vi "Init Control.vi"(5 "Group":refnum<class "Group DBL.lvclass">, 6 "Period ms":i64, 7 "VolatusAPI":refnum<class "VolatusAPI.lvclass">, 8 "error in (no error)":errorcluster, 9 "Control MsgQ":refnum<class "MessageQ.lvclass">, 10 "Config Element":refnum<class "Config Element.lvclass">, 11 "Valve in":refnum<class "LimitControl.lvclass">) -> (0 "error out":errorcluster, 3 "Valve out":refnum<class "LimitControl.lvclass">)   [LabVIEW 2020, in "VolatusControl.lvlib" / "LimitControl.lvclass"]
uses:
  LimitControl.lvclass
  lv-cdm/CDM-Config/Config Element/Config Element.lvclass
  Volatus/VolatusAPI/VolatusAPI.lvclass
  Volatus/MessageQ/MessageQ.lvclass
  lv-vecto/Vecto/Group DBL/Group DBL.lvclass
  C:/dev/lv20CE/relink/lv-vecto/Vecto/Group/Group.lvclass
  PV Calc.ctl
  LimitControl.lvclass/LimitControl.ctl
  lv-vecto/Vecto/Group/Group.lvclass
  VolatusControl.lvlib
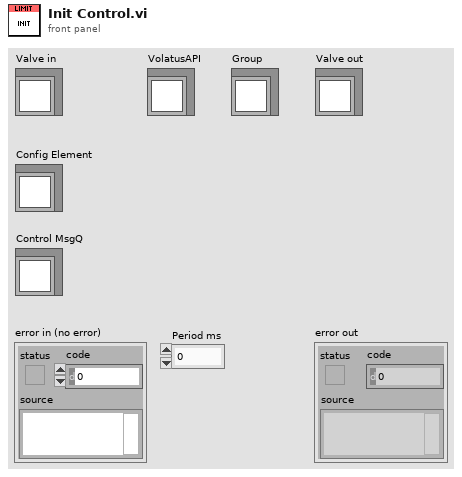
[diagram p1: front panel]
types:
  T1 = typedef "VolatusControl.lvlib/LimitControl.lvclass/PV Calc.ctl" = enum16{"Average", "Median"}
  T2 = typedef "CDM-Config.lvlib/Value Type.ctl" = enum16{"String", "Number", "Bool", "Object", "Array"}
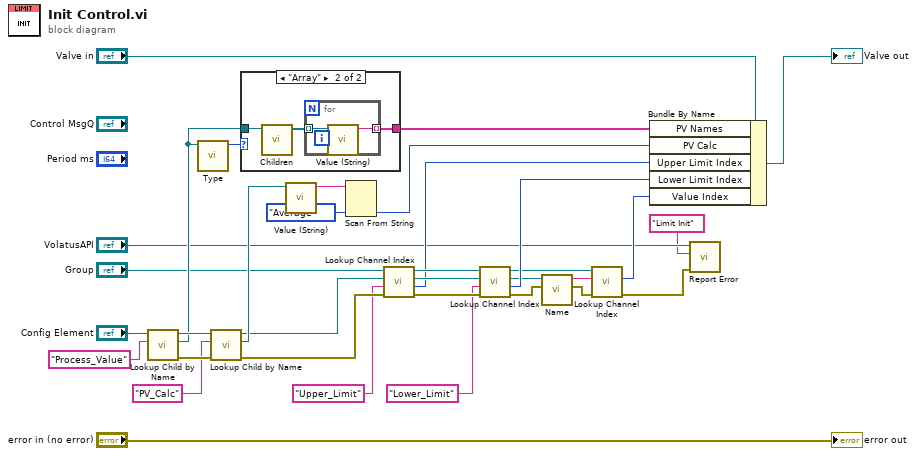
[diagram p0: block diagram]
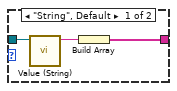
[diagram p2: hidden frame]
diagram:
  n1 = call "Lookup Child by Name.vi"("Name"="Process_Value", "Config Element in"="Config Element") -> ("error out"=w19:errorcluster, "Child"=w26:refnum<class "Config Element.lvclass">, "Config Element out"=w28:refnum<class "Config Element.lvclass">)  [unwired: 6 in, 1 out]
  n2 = call "Type.vi"("Config Element in"=w26) -> ("Value Type"=w27:T2)  [unwired: 9 in, 1 out]
  n3 = call "Lookup Child by Name.vi"("error in (no error)"=w19, "Name"="PV_Calc", "Config Element in"=w28) -> ("error out"=w33:errorcluster, "Child"=w24:refnum<class "Config Element.lvclass">, "Config Element out"=w15:refnum<class "Config Element.lvclass">)  [unwired: 5 in, 1 out]
  n4 = case shown="\"Array\"" w27 {
    tunnel: w26 -> [w37 w40]
    tunnel: [w35 w38] -> w21
    frame "String", Default {
      n5 = call "Value (String).vi"("Config Element in"=w37) -> ("String Value"=w36:string)  [unwired: 9 in, 1 out]
      n6 = Build Array(w36) -> (w35:string[])
    }
    frame "Array" {
      n7 = call "Children.vi"("Config Element in"=w40) -> ("Elements"=w39:refnum<class "Config Element.lvclass">[])  [unwired: 9 in, 1 out]
      n8 = for {
        tunnel: w39 -> [w42] mode=indexing
        tunnel: [w41] -> w38 mode=indexing
        n9 = call "Value (String).vi"("Config Element in"=w42) -> ("String Value"=w41:string)  [unwired: 9 in, 1 out]
      }
    }
  }
  n10 = call "Value (String).vi"("Config Element in"=w24) -> ("String Value"=w25:string)  [unwired: 9 in, 1 out]
  n11 = Scan From String(input string=w25, default 1=PV_Calc."Average" ("PV Calc")) -> (output 1=w20:T1)  [unwired: 3 in, 3 out]
  n12 = call "Lookup Channel Index.vi"("error in (no error)"=w33, "Meta Value"="Upper_Limit" ("Name"), "Config Element in"=w15, "Group in"="Group") -> ("error out"=w34:errorcluster, "Index"=w11:i32, "Config Element"=w13:refnum<class "Config Element.lvclass">, "Group"=w14:refnum<class "Group DBL.lvclass">)  [unwired: 4 in]
  n13 = call "Lookup Channel Index.vi"("error in (no error)"=w34, "Meta Value"="Lower_Limit" ("Name"), "Config Element in"=w13, "Group in"=w14) -> ("error out"=w8:errorcluster, "Index"=w10:i32, "Config Element"=w9:refnum<class "Config Element.lvclass">, "Group"=w5:refnum<class "Group DBL.lvclass">)  [unwired: 4 in]
  n14 = call "Name.vi"("error in (no error)"=w8, "Config Element in"=w9) -> ("error out"=w6:errorcluster, "Name"=w7:string)  [unwired: 8 in]
  n15 = call "Lookup Channel Index.vi"("error in (no error)"=w6, "Channel Name"=w7, "GroupAbstract in"=w5) -> ("error out"=w2:errorcluster, "Index"=w4:i32)  [unwired: 6 in, 1 out]
  n16 = Bundle By Name(cluster="Valve in", "PV Names"=w21, "PV Calc"=w20, "Upper Limit Index"=w11, "Lower Limit Index"=w10, "Value Index"=w4) -> (→"Valve out":refnum<class "LimitControl.lvclass">)
  n17 = call "Report Error.vi"("error in (no error)"=w2, "Context"="Limit Init", "VolatusAPI in"="VolatusAPI") -> ()  [unwired: 7 in, 2 out]
  "error out" <- "error in (no error)"
